vi "BuildCall.vi"(7 "PythonConverter_BD in":refnum<class "PyConvBD.lvclass">, 8 "error in":errorcluster, 11 "Function in":refnum<class "GrowableFunction.lvclass">) -> (0 "error out":errorcluster, 3 "Function out":refnum<class "GrowableFunction.lvclass">, 5 "PythonConverter_BD out":refnum<class "PyConvBD.lvclass">)   [LabVIEW 2014, in "GrowableFunction.lvclass"]
uses:
  GrowableFunction.lvclass
  Python/Parsing/Classes/PythonFunction/PythonFunction.lvclass
  Python/PythonConverter_BD/PyConvBD.lvclass
  Python/PythonConverter_BD/TypeDefs/NodeCall_TD.ctl
  Python/Parsing/Python Functions.lvlib
  Python/Parsing/ListTypesTD.ctl
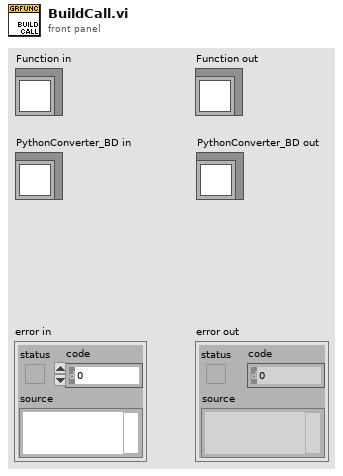
[diagram p1: front panel]
types:
  T1 = typedef "Python Functions.lvlib/ListTypesTD.ctl" = enum16{"list", "tuple", "parameter list", "output list"}
  T2 = typedef "NodeCall_TD.ctl" = cluster{"call":string, "collect":string, "Threaded":bool, "branches":string[]}
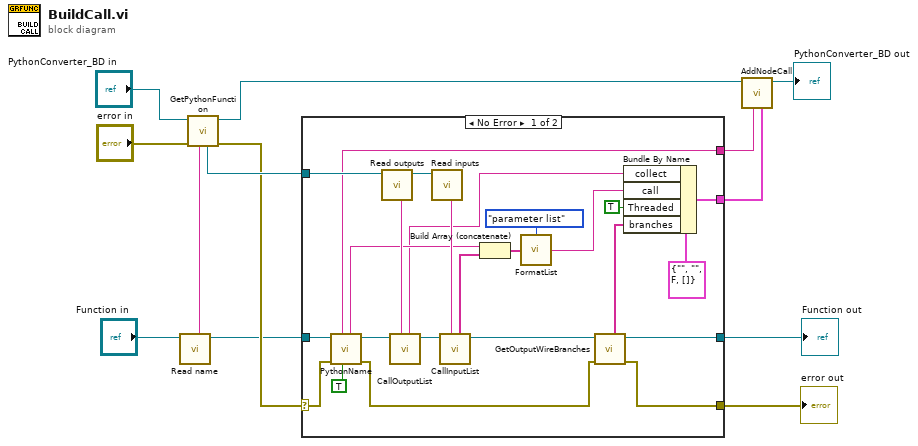
[diagram p0: block diagram]
diagram:
  n1 = call-dynamic "Read name.vi"("Node in"="Function in") -> ("Node out"=w3:refnum<class "GrowableFunction.lvclass">, "name"=w4:string)  [unwired: 7 in]
  n2 = call "GetPythonFunction.vi"("function name"=w4, "error in"="error in", "PythonConverter_BD in"="PythonConverter_BD in") -> ("error out"=w10:errorcluster, "PythonConverter_BD out"=w7:refnum<class "PyConvBD.lvclass">, "Python function"=w11:refnum<class "PythonFunction.lvclass">)  [unwired: 4 in]
  n3 = case shown="No Error" w10 {
    selector: w10 -> [w33 w39]
    tunnel: [w14 w39] -> w13
    tunnel: w3 -> [w32 w38]
    tunnel: w11 -> [w35 _]
    tunnel: [w31 _] -> w6
    tunnel: [w17 w38] -> w2
    tunnel: [w23 _] -> w1
    frame No Error {
      n4 = call-dynamic "PythonName.vi"("add self"=TRUE, "error in"=w33, "Node in"=w32) -> ("error out"=w15:errorcluster, "Node out"=w28:refnum<class "GrowableFunction.lvclass">, "name"=w30:string, "UID"=w31:string)  [unwired: 5 in]
      n5 = call "Read outputs.vi"("PythonFunction in"=w35) -> ("PythonFunction out"=w34:refnum<class "PythonFunction.lvclass">, "outputs"=w37:string)  [unwired: 7 in]
      n6 = call "CallOutputList.vi"("list"=w37, "Function in"=w28) -> ("Function out"=w27:refnum<class "GrowableFunction.lvclass">, "call outputs"=w22:string)  [unwired: 6 in]
      n7 = call "Read inputs.vi"("PythonFunction in"=w34) -> ("inputs"=w36:string)  [unwired: 7 in, 1 out]
      n8 = call "CallInputList.vi"("list"=w36, "Function in"=w27) -> ("Function out"=w18:refnum<class "GrowableFunction.lvclass">, "call inputs"=w29:string[])  [unwired: 6 in]
      n9 = Build Array (concatenate)(w30, w29) -> (w20:string[])
      n10 = call "FormatList.vi"("values"=w20, "type"=ListTypesTD."parameter list") -> ("python object"=w19:string)
      n11 = call-dynamic "GetOutputWireBranches.vi"("error in"=w15, "Node in"=w18) -> ("error out"=w14:errorcluster, "Node out"=w17:refnum<class "GrowableFunction.lvclass">, "branches"=w16:string[])  [unwired: 5 in]
      n12 = Bundle By Name(cluster=T2 {"call"="", "collect"="", "Threaded"=FALSE, "branches"=[]} ("call"), "collect"=w22, "call"=w19, "Threaded"=TRUE, "branches"=w16) -> (w23:T2)
    }
    frame Error {
    }
  }
  "error out" <- w13
  "Function out" <- w2
  n13 = call "AddNodeCall.vi"("call"=w1, "name"=w6, "PythonConverter_BD in"=w7) -> ("PythonConverter_BD out"=→"PythonConverter_BD out":refnum<class "PyConvBD.lvclass">)  [unwired: 5 in, 1 out]
